vi "Wait_for_field_stable.vi"(7 "Magnet PS":u16(ring) items=["Resistive Magnet", "SCM"], 8 "error in (no error)":errorcluster, 10 "Message_command in":T2, 11 "Command_Queue":T3) -> (0 "error out":errorcluster, 2 "Message_command out":T2)   [LabVIEW 2019]
uses:
  Command_Queue.ctl
  Command_Message.ctl
panel:
  out "notify warning":bool
  out "Initial Time":timestamp
  out "measured rate (T/min)":dbl
  out "PS status":T1(ring)=enum."Ramping to programmed field "
  in  "email warning?":bool=TRUE
  out "error indicator":bool
  in  "check ramping status":bool=TRUE
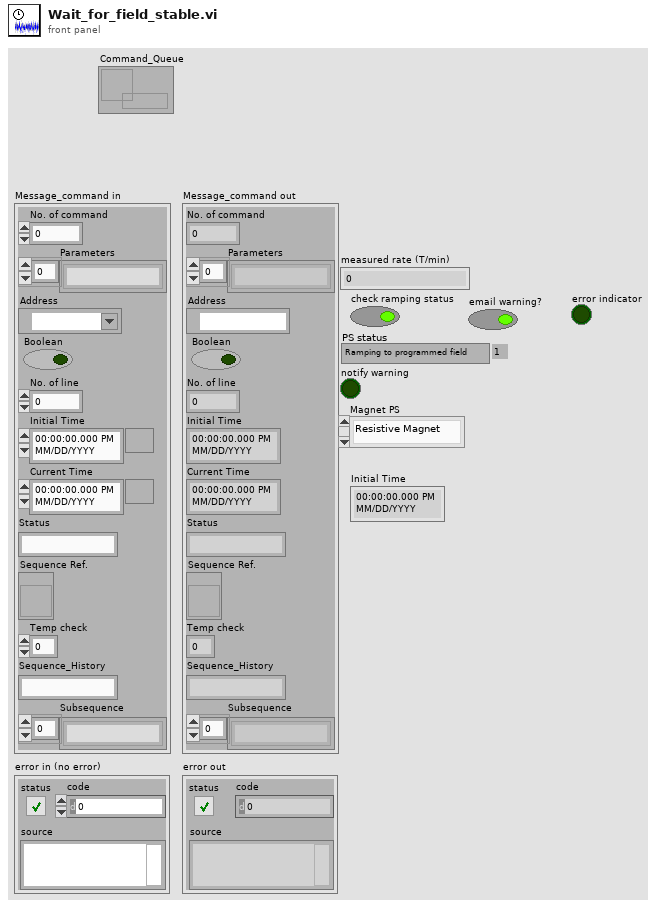
[diagram p1: front panel]
types:
  T1 = enum16{"No Response", "Ramping to programmed field ", "Holding at programmed field", "Paused", "Ramp Manual Up", "Ramp Manual Down", "Ramping to Zero", "QUENCH", "Heating Persistence Switch", "At Zero Current"}
  T2 = typedef "Command_Message.ctl" = cluster{"No. of command":i32, "Parameters":string[], "Address":refnum<visa-resource-name>, "Boolean":bool, "No. of line":i32, "Initial Time":timestamp, "Current Time":timestamp, "Status":string, "Sequence Ref.":refnum<vi>, "Temp check":i32, "Sequence_History":string, "Subsequence":string[]}
  T3 = typedef "Command_Queue.ctl" = refnum<queue>
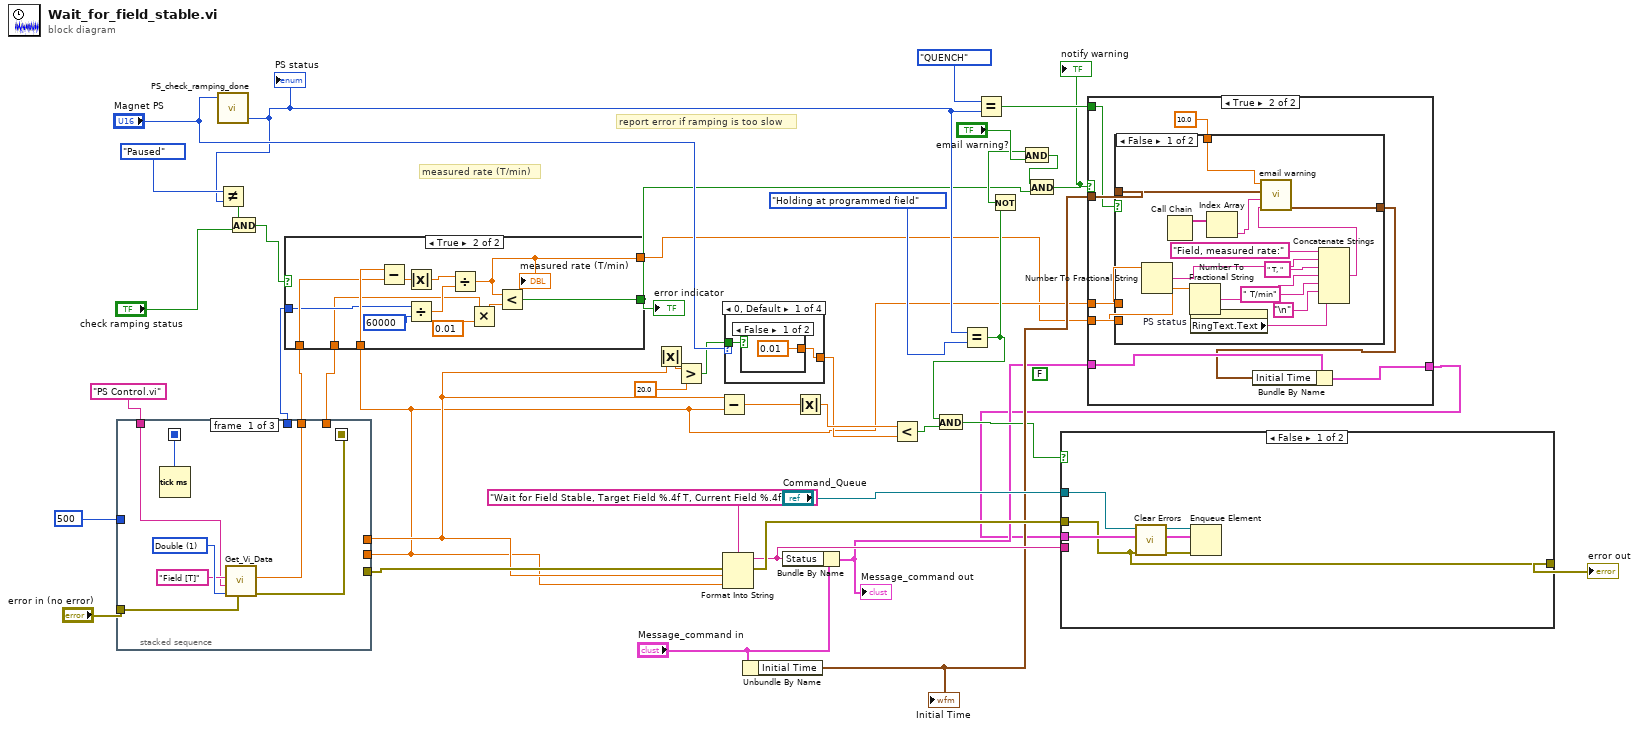
[diagram p0: block diagram]
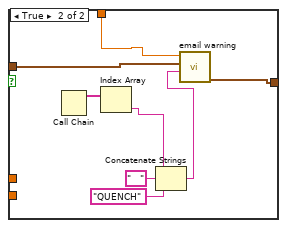
[diagram p3: hidden frame]
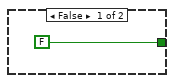
[diagram p4: hidden frame]
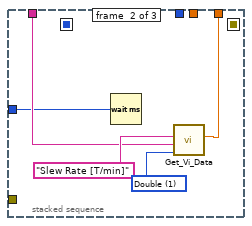
[diagram p5: hidden frame]
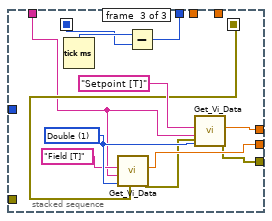
[diagram p6: hidden frame]
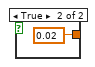
[diagram p7: hidden frame]
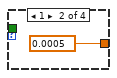
[diagram p8: hidden frame]
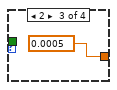
[diagram p9: hidden frame]
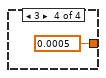
[diagram p10: hidden frame]
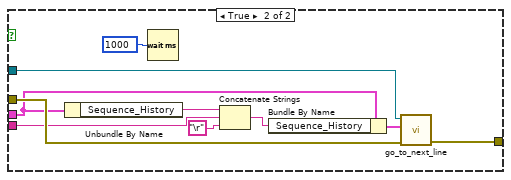
[diagram p11: hidden frame]
diagram:
  (unwired) FALSE ("x .or. y?")
  # "report error if ramping is too slow"
  # "measured rate (T/min)"
  n1 = stacked-sequence {
    seq-local: [w45 _ _] -> [_ _ w59]
    seq-local: [w43 _ _] -> [_ _ w55]
    tunnel: [_ _ w66] -> w2
    tunnel: [_ _ w65] -> w36
    tunnel: "error in (no error)" -> [w47 _ _]
    tunnel: [_ _ w60] -> w30
    tunnel: "PS Control.vi" ("VI name") -> [w46 w52 w58]
    tunnel: [_ w51 _] -> w24
    tunnel: [w44 _ _] -> w23
    tunnel: u32 500 ("milliseconds to wait") -> [_ w50 _]
    tunnel: [_ _ w57] -> w18
    frame #0 {
      w49 = u16 1 items=["String", "Double", "Boolean", "Variant"] ("Data Type")
      n2 = Tick Count (ms)() -> (millisecond timer value=w43:u32)
      n3 = call "Get_Vi_Data.vi"("error in (no error) 2"=w47, "Data Type"=w49, "VI name"=w46, "Control Name"="Field [T]") -> ("error out"=w45:errorcluster, "Data (Double)"=w44:dbl)  [unwired: 3 in, 3 out]
    }
    frame #1 {
      w54 = u16 1 items=["String", "Double", "Boolean", "Variant"] ("Data Type")
      n4 = Wait (ms)(milliseconds to wait=w50) -> ()  [unwired: 1 out]
      n5 = call "Get_Vi_Data.vi"("Data Type"=w54, "VI name"=w52, "Control Name"="Slew Rate [T/min]" ("VI name")) -> ("Data (Double)"=w51:dbl)  [unwired: 4 in, 4 out]
    }
    frame #2 {
      w64 = u16 1 items=["String", "Double", "Boolean", "Variant"] ("Data Type")
      n6 = Tick Count (ms)() -> (millisecond timer value=w56:u32)
      n7 = call "Get_Vi_Data.vi"("error in (no error) 2"=w59, "Data Type"=w64, "VI name"=w58, "Control Name"="Field [T]") -> ("error out"=w62:errorcluster, "Data (Double)"=w66:dbl)  [unwired: 3 in, 3 out]
      n8 = Subtract(x=w56, y=w55) -> (x-y=w57:u32)
      n9 = call "Get_Vi_Data.vi"("error in (no error) 2"=w62, "Data Type"=w64, "VI name"=w58, "Control Name"="Setpoint [T]") -> ("error out"=w65:errorcluster, "Data (Double)"=w60:dbl)  [unwired: 3 in, 3 out]
    }
  }
  n10 = call "PS_check_ramping_done.vi"("Magnet PS"="Magnet PS") -> ("PS status"=w15:T1)  [unwired: 1 in]
  "PS status" <- w15
  n11 = Not Equal?(x=T1."Paused" ("PS status"), y=w15) -> (x != y?=w21:bool)
  n12 = And(x=w21, y="check ramping status") -> (x .and. y?=w20:bool)
  n13 = case shown="True" w20 {
    tunnel: w2 -> [_ w79]
    tunnel: w24 -> [_ w72]
    tunnel: w23 -> [_ w76]
    tunnel: w18 -> [_ w75]
    tunnel: [FALSE w69] -> w4
    tunnel: [_ w68] -> w1
    frame False {
    }
    frame True {
      n14 = Subtract(x=w79, y=w76) -> (x-y=w78:dbl)
      n15 = Absolute Value(x=w78) -> (abs(x)=w77:dbl)
      n16 = Divide(x=w75, y=u32 60000) -> (x/y=w73:dbl)
      n17 = Divide(x=w77, y=w73) -> (x/y=w68:dbl)
      "measured rate (T/min)" <- w68
      n18 = Multiply(x=w72, y=0.01) -> (x*y=w71:dbl)
      n19 = Less?(x=w68, y=w71) -> (x < y?=w69:bool)
    }
  }
  "error indicator" <- w4
  n20 = Absolute Value(x=w30) -> (abs(x)=w29:dbl)
  n21 = Greater?(x=w29, y=20.0) -> (0:w27:bool)
  n22 = Subtract(x=w30, y=w2) -> (x-y=w42:dbl)
  n23 = Format Into String(format string="Wait for Field Stable, Target Field %.4f T, Current Field %.4f T" ("Status"), error in=w36, w30, w2) -> (resulting string=w35:string, error out=w37:errorcluster)  [unwired: 1 in]
  n24 = case shown="0, Default" "Magnet PS" {
    tunnel: [w81 0.0005 ("y") 0.0005 ("y") 0.0005 ("y")] -> w31
    tunnel: w27 -> [w80 _ _ _]
    frame 0, Default {
      n25 = case shown="False" w80 {
        tunnel: [0.01 ("y") 0.02 ("y")] -> w81
        frame False {
        }
        frame True {
        }
      }
    }
    frame 1 {
    }
    frame 2 {
    }
    frame 3 {
    }
  }
  n26 = Unbundle By Name("Message_command in") -> ("Initial Time"=w17:timestamp)
  "Initial Time" <- w17
  n27 = Bundle By Name(cluster="Message_command in", "Status"=w35) -> (w8:T2)
  "Message_command out" <- w8
  n28 = Absolute Value(x=w42) -> (abs(x)=w41:dbl)
  n29 = Less?(x=w41, y=w31) -> (x < y?=w33:bool)
  n30 = Equal?(x=w15, y=T1."Holding at programmed field" ("PS status")) -> (x = y?=w9:bool)
  n31 = And(x=w9, y=w33) -> (x .and. y?=w10:bool)
  n32 = Equal?(x=T1."QUENCH" ("PS status"), y=w15) -> (x = y?=w13:bool)
  n33 = Not(x=w9) -> (.not. x?=w6:bool)
  n34 = And(x=w6, y="email warning?") -> (x .and. y?=w5:bool)
  n35 = And(x=w5, y=w4) -> (x .and. y?=w3:bool)
  "notify warning" <- w3
  n36 = case shown="True" w3 {
    tunnel: w17 -> [_ w95]
    tunnel: w13 -> [_ w94]
    tunnel: w8 -> [w87 w93]
    tunnel: [w87 w92] -> w7
    tunnel: w2 -> [_ w89]
    tunnel: w1 -> [_ w88]
    frame False {
    }
    frame True {
      n37 = case shown="False" w94 {
        tunnel: w95 -> [w110 w118]
        tunnel: [w107 w112] -> w91
        tunnel: 10.0 ("email interval (min)") -> [w106 w111]
        tunnel: w89 -> [w104 _]
        tunnel: w88 -> [w101 _]
        frame False {
          n38 = Number To Fractional String(number=w104) -> (F-format string=w103:string)  [unwired: 3 in]
          n39 = Call Chain() -> (call chain=w109:string[])
          n40 = Number To Fractional String(number=w101) -> (F-format string=w100:string)  [unwired: 3 in]
          n41 = property on="PS status" class="Enum (strict)"() -> ("RingText.Text"=w96:string)  [unwired: 2 in, 2 out]
          n42 = Index Array(array=w109) -> (element=w108:string)  [unwired: 1 in]
          n43 = Concatenate Strings("Field, measured rate:" ("string"), w103, " T, " ("string"), w100, " T/min" ("string"), "\n", w96) -> (w98:string)
          n44 = call "email warning.vi"("Message"=w98, "running VI"=w108, "Initial"=w110, "email interval (min)"=w106) -> ("notified timestamp"=w107:timestamp)  [unwired: 7 in]
        }
        frame True {
          n45 = Call Chain() -> (call chain=w117:string[])
          n46 = Index Array(array=w117) -> (element=w116:string)  [unwired: 1 in]
          n47 = Concatenate Strings(w116, "   " ("string"), "QUENCH" ("string")) -> (w113:string)
          n48 = call "email warning.vi"("running VI"=w113, "Initial"=w118, "email interval (min)"=w111) -> ("notified timestamp"=w112:timestamp)  [unwired: 8 in]
        }
      }
      n49 = Bundle By Name(cluster=w93, "Initial Time"=w91) -> (w92:T2)
    }
  }
  n50 = case shown="False" w10 {
    tunnel: w37 -> [w119 w131]
    tunnel: w7 -> [w122 w128]
    tunnel: "Command_Queue" -> [w121 w132]
    tunnel: [w119 w130] -> w39
    tunnel: w35 -> [_ w126]
    frame False {
      n51 = call <vilib>:"Clear Errors.vi"("error in (no error)"=w119) -> ("error out"=w120:errorcluster)  [unwired: 5 in, 1 out]
      n52 = Enqueue Element(queue=w121, element=w122, error in (no error)=w120) -> ()  [unwired: 1 in, 3 out]
    }
    frame True {
      n53 = Unbundle By Name(w128) -> ("Sequence_History"=w127:string)
      n54 = Wait (ms)(milliseconds to wait=u32 1000) -> ()  [unwired: 1 out]
      n55 = Concatenate Strings(w127, w126, "\r") -> (w124:string)
      n56 = Bundle By Name(cluster=w128, "Sequence_History"=w124) -> (w123:T2)
      n57 = call "go_to_next_line.vi"("error in (no error)"=w131, "Message_command in"=w123, "Command Queue in"=w132) -> ("error out"=w130:errorcluster)  [unwired: 7 in, 1 out]
    }
  }
  "error out" <- w39
